vi "Configure Protocol Settings Dual Channel.vi"(8 "error in":errorcluster, 11 "Protocol settings":T2={"Protocol capture resource name"="", "Data line"=0, "Channel"="", "Clock rate"=12288000, "Number of words"=19200, "Sensitivity"=0.34762, "Frame sync edge for channel 0"=enum."Falling", "Channel count per frame"=2, "Channel length"=32, "Bit depth"=24, "Channel 0 offset"=1, "Endianness"=enum."MSB First", "Data justification"=enum."Left Justified", "Frame length"=64, "Frame sync pulse width"=32, "Bit clock edge sync"=enum."Falling"}) -> (0 "error out":errorcluster, 3 "PCM input task out":T1)   [LabVIEW 2021, in "Audio ADC Shared.lvlib"]
uses:
  Audio ADC Shared.lvlib
  controls/Protocol Settings Dual Channel.ctl
  <vilib>/PDM Acquisition Toolkit/host/Classes/Tasks/PCM Input/Controls/DVR PCM Input Task.ctl
  <vilib>/PDM Acquisition Toolkit/host/Classes/Tasks/PCM Input/PCM Input Task.lvclass
  <vilib>/PDM Acquisition Toolkit/host/Classes/Tasks/PDM Tasks/Controls/Acquisition Mode.ctl
  <vilib>/PDM Acquisition Toolkit/host/Classes/Session/Controls/Logic Levels.ctl
  <vilib>/PDM Acquisition Toolkit/shared/controls/PCM Data Format Configuration.ctl
  <vilib>/PDM Acquisition Toolkit/shared/controls/Digital Edge.ctl
  <vilib>/PDM Acquisition Toolkit/shared/controls/PCM Bit Endianness.ctl
  <vilib>/PDM Acquisition Toolkit/shared/controls/PCM Data Justification.ctl
  <vilib>/PDM Acquisition Toolkit/shared/controls/PCM Frame Sync Control.ctl
  <vilib>/PDM Acquisition Toolkit/host/API/Public/Create Tasks/Create PCM Input Task.vi
  <vilib>/PDM Acquisition Toolkit/host/API/Public/Configure/Timing/Configure Timing - PCM Input Slave.vi
  <vilib>/PDM Acquisition Toolkit/host/API/Public/Configure/PDM Channel/Configure Microphone Sensitivity FSPA - PCM Input Task.vi
  <vilib>/PDM Acquisition Toolkit/host/API/PDM Acquisition Toolkit.lvlib
  <vilib>/PDM Acquisition Toolkit/host/Classes/Tasks/PDM Tasks/PDM Task.lvclass
  <vilib>/PDM Acquisition Toolkit/host/Classes/Session/DecoderSession.lvclass
  <vilib>/PDM Acquisition Toolkit/shared/PDM Shared.lvlib
  controls/Audio ADC Controls.lvlib
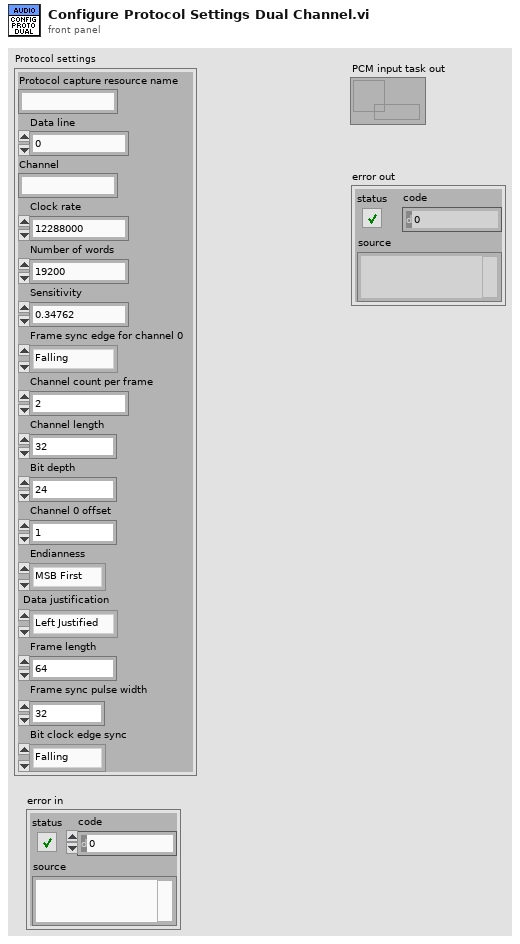
[diagram p1: front panel]
types:
  T1 = typedef "PDM Acquisition Class Library.lvlib/PCM Input Task.lvclass/DVR PCM Input Task.ctl" = refnum<data-value>
  T2 = typedef "Audio ADC Controls.lvlib/Protocol Settings Dual Channel.ctl" = cluster{"Protocol capture resource name":string, "Data line":u16, "Channel":string, "Clock rate":u32, "Number of words":i32, "Sensitivity":dbl, "Frame sync edge for channel 0":enum32{"Rising", "Falling"}, "Channel count per frame":u8, "Channel length":u16, "Bit depth":u8, "Channel 0 offset":u16, "Endianness":enum32{"MSB First", "LSB First"}, "Data justification":enum32{"Left Justified", "Right Justified"}, "Frame length":u16, "Frame sync pulse width":u16, "Bit clock edge sync":enum32{"Rising", "Falling"}}
  T3 = typedef "PDM Shared.lvlib/PCM Frame Sync Control.ctl" = cluster{"Frame Length":u16, "Frame Sync Pulse Width":u16, "Bit Clock Edge  Sync":T4}
  T4 = typedef "PDM Shared.lvlib/Digital Edge.ctl" = enum8{"Rising", "Falling"}
  T5 = typedef "PDM Shared.lvlib/PCM Data Format Configuration.ctl" = cluster{"Frame Sync Edge for Channel 0":T4, "Channel Count Per Frame":u8, "Channel Length":u16, "Bit Depth":u8, "Channel 0 Offset":u16, "Endianness":T6, "Data Justification":T7}
  T6 = typedef "PDM Shared.lvlib/PCM Bit Endianness.ctl" = enum16{"MSB First", "LSB First"}
  T7 = typedef "PDM Shared.lvlib/PCM Data Justification.ctl" = enum16{"Left Justified", "Right Justified"}
  T8 = typedef "PDM Acquisition Class Library.lvlib/DecoderSession.lvclass/Logic Levels.ctl" = enum16{"3.3 V", "1.8 V", "1.2 V"}
  T9 = typedef "PDM Acquisition Class Library.lvlib/PDM Task.lvclass/Acquisition Mode.ctl" = enum16{"Finite", "Continuous"}
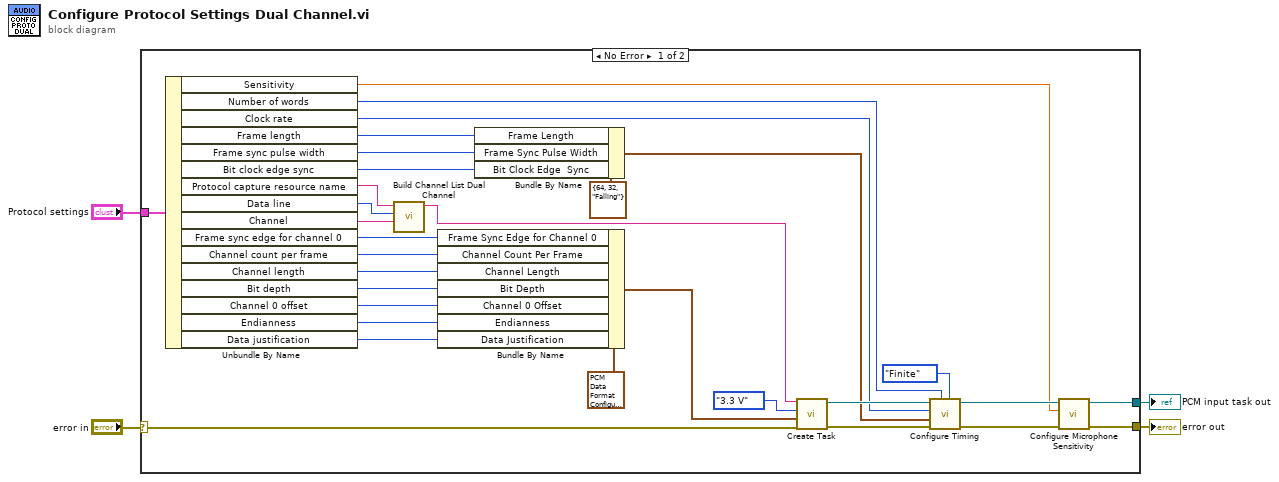
[diagram p0: block diagram]
diagram:
  n1 = case shown="No Error" "error in" {
    selector: "error in" -> [w10 w36]
    tunnel: "Protocol settings" -> [w35 _]
    tunnel: [w6 _] -> w2
    tunnel: [w5 w36] -> w1
    frame No Error {
      n2 = Unbundle By Name(w35) -> ("Sensitivity"=w23:dbl, "Number of words"=w22:i32, "Clock rate"=w21:u32, "Frame length"=w20:u16, "Frame sync pulse width"=w19:u16, "Bit clock edge sync"=w18:enum32{"Rising", "Falling"}, "Protocol capture resource name"=w9:string, "Data line"=w8:u16, "Channel"=w7:string, "Frame sync edge for channel 0"=w17:enum32{"Rising", "Falling"}, "Channel count per frame"=w16:u8, "Channel length"=w15:u16, "Bit depth"=w14:u8, "Channel 0 offset"=w13:u16, "Endianness"=w12:enum32{"MSB First", "LSB First"}, "Data justification"=w11:enum32{"Left Justified", "Right Justified"})
      n3 = call "Build Channel List Dual Channel.vi"("Channel"=w7, "Data line"=w8, "Protocol capture resource name"=w9) -> ("String"=w24:string)  [unwired: 8 in]
      n4 = Bundle By Name(cluster=T5 {"Frame Sync Edge for Channel 0"=enum."Falling", "Channel Count Per Frame"=2, "Channel Length"=32, "Bit Depth"=24, "Channel 0 Offset"=1, "Endianness"=enum."MSB First", "Data Justification"=enum."Left Justified"} ("PCM data configuration"), "Frame Sync Edge for Channel 0"=w17, "Channel Count Per Frame"=w16, "Channel Length"=w15, "Bit Depth"=w14, "Channel 0 Offset"=w13, "Endianness"=w12, "Data Justification"=w11) -> (w29:T5)
      n5 = Bundle By Name(cluster=T3 {"Frame Length"=64, "Frame Sync Pulse Width"=32, "Bit Clock Edge  Sync"=enum."Falling"} ("Frame Sync Clock Control"), "Frame Length"=w20, "Frame Sync Pulse Width"=w19, "Bit Clock Edge  Sync"=w18) -> (w27:T3)
      n6 = call-poly <vilib>:"Create Task.vi"("error in"=w10, "PCM data configuration"=w29, "logic level"=Logic_Levels."3.3 V", "channel list"=w24) -> ("error out"=w33:errorcluster, "PCM input task out"=w34:T1)  [unwired: 6 in]
      n7 = call-poly <vilib>:"Configure Timing.vi"("acquisition mode"=Acquisition_Mode."Finite", "Frame Sync Clock Control"=w27, "number of words per channel"=w22, "error in"=w33, "Bit Clock rate"=w21, "PCM input task in"=w34) -> ("error out"=w25:errorcluster, "PCM input task out"=w26:T1)  [unwired: 4 in]
      n8 = call-poly <vilib>:"Configure Microphone Sensitivity.vi"("error in"=w25, "microphone sensitivity (FS/Pa)"=w23, "PCM input task in"=w26) -> ("error out"=w5:errorcluster, "PCM input task out"=w6:T1)  [unwired: 7 in]
    }
    frame Error {
    }
  }
  "PCM input task out" <- w2
  "error out" <- w1
